vi "ControlDisengageSystems (1).vi"   [LabVIEW 2017]
doc: "Output FALSE to solenoids controlling Levitiation, Suspension, and Magnetic Braking."
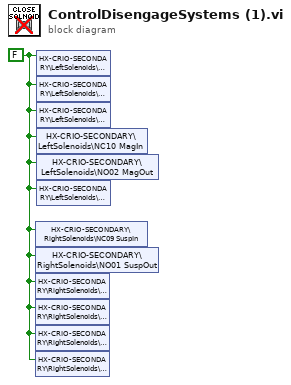
[diagram p0: block diagram]
diagram:
  w1 = FALSE
  n1 = shared-variable "HX-CRIO-SECONDARY\\RightSolenoids\\NC09 SuspIn"(w1) -> ()  [unwired: 1 in, 1 out]
  n2 = shared-variable "HX-CRIO-SECONDARY\\RightSolenoids\\NO01 SuspOut"(w1) -> ()  [unwired: 1 in, 1 out]
  n3 = shared-variable "HX-CRIO-SECONDARY\\RightSolenoids\\NC08"(w1) -> ()  [unwired: 1 in, 1 out]
  n4 = shared-variable "HX-CRIO-SECONDARY\\RightSolenoids\\NC05"(w1) -> ()  [unwired: 1 in, 1 out]
  n5 = shared-variable "HX-CRIO-SECONDARY\\RightSolenoids\\NC06"(w1) -> ()  [unwired: 1 in, 1 out]
  n6 = shared-variable "HX-CRIO-SECONDARY\\RightSolenoids\\NC07"(w1) -> ()  [unwired: 1 in, 1 out]
  n7 = shared-variable "HX-CRIO-SECONDARY\\LeftSolenoids\\NC03"(w1) -> ()  [unwired: 1 in, 1 out]
  n8 = shared-variable "HX-CRIO-SECONDARY\\LeftSolenoids\\NC04"(w1) -> ()  [unwired: 1 in, 1 out]
  n9 = shared-variable "HX-CRIO-SECONDARY\\LeftSolenoids\\NC02"(w1) -> ()  [unwired: 1 in, 1 out]
  n10 = shared-variable "HX-CRIO-SECONDARY\\LeftSolenoids\\NC10 MagIn"(w1) -> ()  [unwired: 1 in, 1 out]
  n11 = shared-variable "HX-CRIO-SECONDARY\\LeftSolenoids\\NO02 MagOut"(w1) -> ()  [unwired: 1 in, 1 out]
  n12 = shared-variable "HX-CRIO-SECONDARY\\LeftSolenoids\\NC01"(w1) -> ()  [unwired: 1 in, 1 out]
